vi "Table, Set Column Header Text Bold.vi"(5 "Bold (T)":bool=TRUE, 6 "error in":errorcluster, 9 "Tbl Refnum":refnum<vi>) -> (0 "error out":errorcluster, 3 "Tbl Refnum out":refnum<vi>)   [LabVIEW 2010]
doc: "This function sets table column headers to bold."
uses:
  <vilib>/Utility/miscctls.llb/LVRowAndColumnTypeDef.ctl
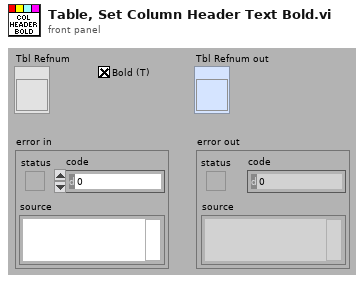
[diagram p1: front panel]
types:
  T1 = typedef "LVRowAndColumnTypeDef.ctl" = cluster{"Row":i32, "Column":i32}
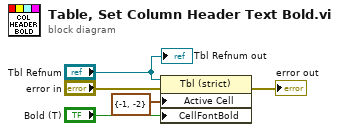
[diagram p0: block diagram]
diagram:
  n1 = property class="Tbl (strict)"(reference="Tbl Refnum", error in="error in", "Active Cell"=T1 {"Row"=-1, "Column"=-2} ("Active Cell:Active Cell"), "CellFontBold"="Bold (T)") -> (error out=→"error out":errorcluster)  [unwired: 1 out]
  "Tbl Refnum out" <- "Tbl Refnum"
